vi "Open-Create-Replace File.vi"(6 "Disable Buffering (F)":bool, 7 "Prompt":refnum<class "UTF-8 String.lvclass">, 8 "error in":errorcluster, 9 "Access (0:read/write)":enum16{"read/write", "read-only", "write-only"}(ring), 10 "Operation (0:open)":T1(ring), 11 "Path (Use Dialog)":refnum<class "UTF-8 Path.lvclass">) -> (0 "error out":errorcluster, 1 "Cancelled":bool, 3 "Refnum out":refnum<file>)   [LabVIEW 2020, in "G-Unicode.lvlib"]
doc: "Opens an existing file, creates a new file, or replaces an existing file, programmatically or interactively using a file dialog box. This function does not work for files inside an LLB."
uses:
  G-Unicode.lvlib
  e07117c9-d87a-4df6-978c-25aa8b1cd0ee.vi
  d3990f92-3b16-4737-ab48-aa5676319d3d.vi
  8c85baee-056b-4e61-8f46-2ccaf65b104b.vi
  Dialog & User Interface/Message Box/Message Box Dialog Type.ctl
  Dialog & User Interface/Message Box/Message Box Icon Type.ctl
  5df6ca1b-9e66-4eda-b70b-79e7b4609640.vi
  d08ebd68-58ab-4e40-b3db-5adaf790fc4e.vi
  Types/UTF-8 Path/UTF-8 Path.lvclass
  Types/UTF-8 String/UTF-8 String.lvclass
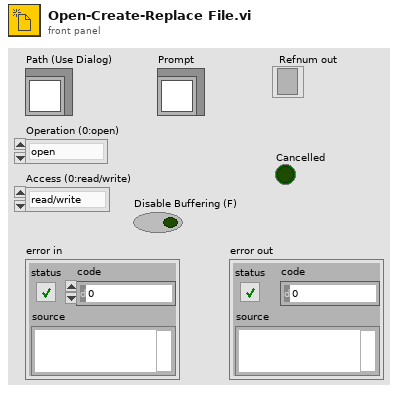
[diagram p1: front panel]
types:
  T1 = enum16{"open", "replace", "create", "open or create", "replace or create", "replace or create with confirmation"}
  T2 = typedef "G-Unicode.lvlib/Message Box Icon Type.ctl" = enum16{"Info", "Warning", "Error", "Question"}
  T3 = typedef "G-Unicode.lvlib/Message Box Dialog Type.ctl" = enum16{"OK", "OK/Cancel", "Yes/No", "Yes/No/Cancel"}
  T4 = typedef "G-Unicode.lvlib/Message Box Dialog Button.ctl" = enum16{"OK", "Yes", "No", "Cancel"}
  T5 = typedef "G-Unicode.lvlib/Raw UTF-8 Path.ctl" = path
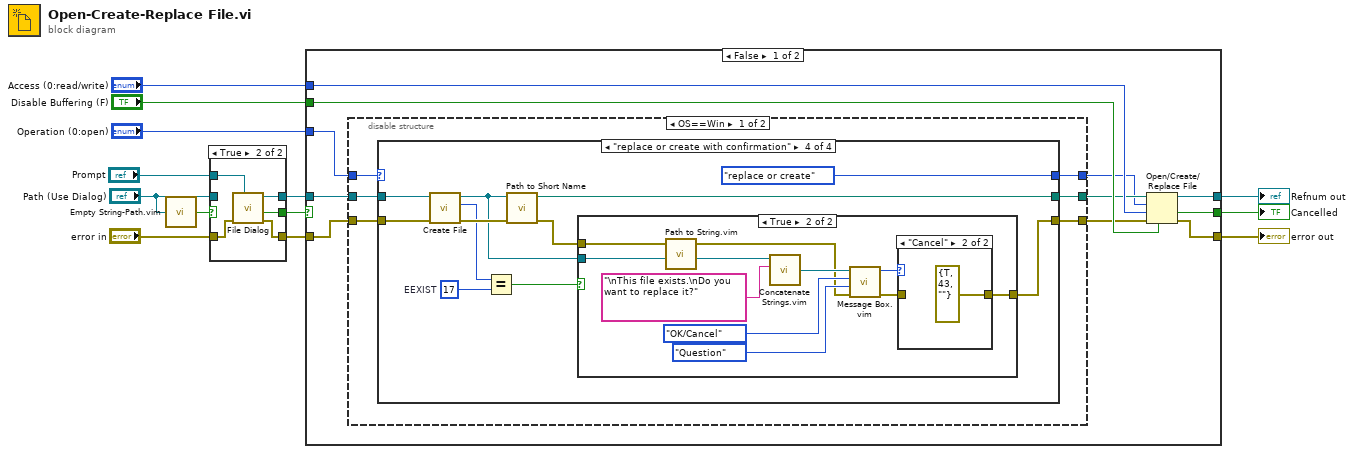
[diagram p0: block diagram]
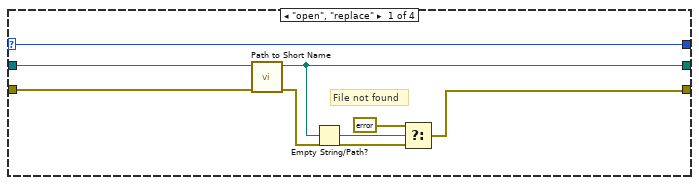
[diagram p2: hidden frame]
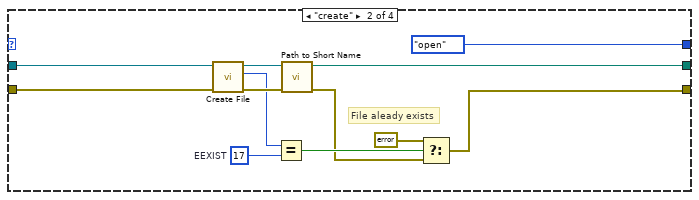
[diagram p3: hidden frame]
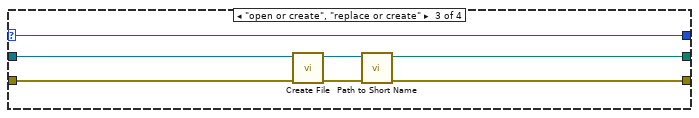
[diagram p4: hidden frame]
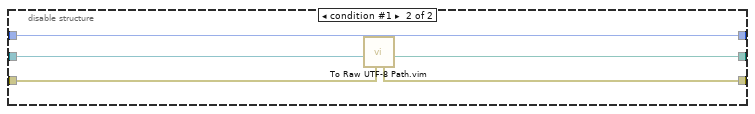
[diagram p7: hidden frame]
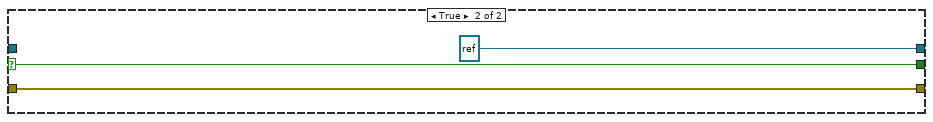
[diagram p8: hidden frame]
diagram:
  n1 = call "Empty String-Path.vim"("String/Path"="Path (Use Dialog)") -> ("Empty?"=w13:bool)
  n2 = case shown="True" w13 {
    selector: w13 -> [w15 _]
    tunnel: [w16 w20] -> w10
    tunnel: "Path (Use Dialog)" -> [w16 _]
    tunnel: "error in" -> [w14 w21]
    tunnel: [w15 w18] -> w9
    tunnel: [w14 w19] -> w8
    tunnel: "Prompt" -> [_ w17]
    frame False {
    }
    frame True {
      n3 = call "File Dialog.vi"("Prompt"=w17, "error in"=w21) -> ("error out"=w19:errorcluster, "Cancelled"=w18:bool, "Selected Path"=w20:refnum<class "UTF-8 Path.lvclass">)  [unwired: 7 in]
    }
  }
  n4 = case shown="False" w9 {
    selector: w9 -> [_ w96]
    tunnel: w10 -> [w26 _]
    tunnel: w8 -> [w25 w97]
    tunnel: [w32 w97] -> w7
    tunnel: [w31 refnum<file> refnum ("refnum out")] -> w6
    tunnel: [w30 w96] -> w5
    tunnel: "Operation (0:open)" -> [w27 _]
    tunnel: "Access (0:read/write)" -> [w29 _]
    tunnel: "Disable Buffering (F)" -> [w28 _]
    frame False {
      n5 = disable-structure shown="OS==Win" {
        disable-tunnel: w27 -> [w38 w92]
        disable-tunnel: w26 -> [w37 w94]
        disable-tunnel: w25 -> [w36 w91]
        disable-tunnel: [w35 w93] -> w24
        disable-tunnel: [w34 w90] -> w23
        disable-tunnel: [w33 w92] -> w22
        frame condition #0 (active) {
          n6 = case shown="\"replace or create with confirmation\"" w38 {
            selector: w38 -> [w39 _ w59 _]
            tunnel: [w42 w54 w60 w73] -> w35
            tunnel: w37 -> [w46 w58 w65 w76]
            tunnel: w36 -> [w45 w57 w64 w75]
            tunnel: [w43 w49 w62 w67] -> w34
            tunnel: [w39 T1."open" ("Operation (0:open)") w59 T1."replace or create" ("Operation (0:open)")] -> w33
            frame "open", "replace" {
              # "File not found"
              n7 = call "Path to Short Name.vi"("error in"=w45, "Path"=w46) -> ("error out"=w41:errorcluster, "LabVIEW Path"=w42:path)  [unwired: 8 in]
              n8 = Empty String/Path?(string/path=w42) -> (empty?=w44:bool)
              n9 = Select(t=errorcluster {"status"=TRUE, "code"=7, "source"=""} ("error constant"), s=w44, f=w41) -> (s? t:f=w43:errorcluster)
            }
            frame "create" {
              w50 = 17  # EEXIST
              # "File aleady exists"
              n10 = call "Create File.vi"("error in"=w57, "Path"=w58) -> ("error out"=w56:errorcluster, "result"=w51:i32, "Path dup"=w55:refnum<class "UTF-8 Path.lvclass">)  [unwired: 7 in]
              n11 = Equal?(x=w51, y=w50) -> (x = y?=w53:bool)
              n12 = call "Path to Short Name.vi"("error in"=w56, "Path"=w55) -> ("error out"=w48:errorcluster, "LabVIEW Path"=w54:path)  [unwired: 8 in]
              n13 = Select(t=errorcluster {"status"=TRUE, "code"=10, "source"=""} ("error constant"), s=w53, f=w48) -> (s? t:f=w49:errorcluster)
            }
            frame "open or create", "replace or create" {
              n14 = call "Create File.vi"("error in"=w64, "Path"=w65) -> ("error out"=w63:errorcluster, "Path dup"=w61:refnum<class "UTF-8 Path.lvclass">)  [unwired: 7 in, 1 out]
              n15 = call "Path to Short Name.vi"("error in"=w63, "Path"=w61) -> ("error out"=w62:errorcluster, "LabVIEW Path"=w60:path)  [unwired: 8 in]
            }
            frame "replace or create with confirmation" {
              w72 = 17  # EEXIST
              n16 = call "Create File.vi"("error in"=w75, "Path"=w76) -> ("error out"=w74:errorcluster, "result"=w71:i32, "Path dup"=w69:refnum<class "UTF-8 Path.lvclass">)  [unwired: 7 in]
              n17 = Equal?(x=w71, y=w72) -> (x = y?=w70:bool)
              n18 = call "Path to Short Name.vi"("error in"=w74, "Path"=w69) -> ("error out"=w68:errorcluster, "LabVIEW Path"=w73:path)  [unwired: 8 in]
              n19 = case shown="True" w70 {
                tunnel: w69 -> [_ w83]
                tunnel: w68 -> [w77 w80]
                tunnel: [w77 w78] -> w67
                frame False {
                }
                frame True {
                  n20 = call "Path to String.vim"("Path"=w83) -> ("String"=w82:refnum<class "UTF-8 String.lvclass">)  [unwired: 9 in, 1 out]
                  n21 = call "Concatenate Strings.vim"("Input 1"="\nThis file exists.\nDo you want to replace it?", "Input 0"=w82) -> ("Concatenated String"=w87:refnum<class "UTF-8 String.lvclass">)  [unwired: 7 in, 1 out]
                  n22 = call "Message Box.vim"("error in"=w80, "Icon Type (Info)"=Message_Box_Icon_Type."Question", "Dialog Type (OK)"=Message_Box_Dialog_Type."OK/Cancel", "Message"=w87) -> ("error out"=w79:errorcluster, "Button"=w81:T4)  [unwired: 6 in]
                  n23 = case shown="\"Cancel\"" w81 {
                    tunnel: w79 -> [w88 _]
                    tunnel: [w88 errorcluster {"status"=TRUE, "code"=43, "source"=""} ("error out")] -> w78
                    frame Default {
                    }
                    frame "Cancel" {
                    }
                  }
                }
              }
            }
          }
        }
        frame condition #1 {
          n24 = call "To Raw UTF-8 Path.vim"("error in"=w91, "Data"=w94) -> ("Raw UTF-8 Path"=w93:T5, "error out"=w90:errorcluster)  [unwired: 8 in]
        }
      }
      n25 = Open/Create/Replace File(file path (use dialog)=w24, error in=w23, operation (0:open)=w22, access (0:read/write)=w29, disable buffering (F)=w28) -> (refnum out=w31:refnum<file>, cancelled=w30:bool, error out=w32:errorcluster)  [unwired: 1 in]
    }
    frame True {
    }
  }
  "error out" <- w7
  "Refnum out" <- w6
  "Cancelled" <- w5
